vi "AIM 664 test Find Disabled Custom Device.vi"(8 "error in":errorcluster, 11 "TestCase in":refnum<class "AIM 664 Scripting.lvclass">) -> (0 "error out":errorcluster, 3 "TestCase out":refnum<class "AIM 664 Scripting.lvclass">)   [LabVIEW 2020, in "AIM 664 Scripting.lvclass"]
uses:
  AIM 664 Scripting.lvclass
  C:/Program Files (x86)/National Instruments/LabVIEW 2020/vi.lib/NI/VeriStand Custom Device Testing Tools/VeriStandScriptingTestCase/VeriStandScriptingTestCase.lvclass
  <vilib>/NI/VeriStand Custom Device Testing Tools/VeriStandScriptingTestCase/VeriStandScriptingTestCase.lvclass/VeriStandScriptingTestCase.ctl
  <vilib>/NI/VeriStand Custom Device Testing Tools/VeriStandScriptingTestCase/Read Target.vi
  NationalInstruments.VeriStand.SystemDefinitionAPI
  <vilib>/addons/_JKI Toolkits/VI Tester/TestCase.llb/TestCase.lvclass
  Scripting/AIM ARINC 664 Scripting.lvlib
  C:/Program Files (x86)/National Instruments/LabVIEW 2020/vi.lib/addons/_JKI Toolkits/VI Tester/TestCase.llb/TestCase.lvclass
  C:/repos/niveristand-aim-arinc664-custom-device/Source/Custom Device Support/Tests/Unit/Scripting/AIM 664 Scripting.lvclass
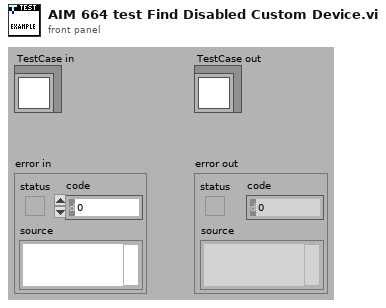
[diagram p1: front panel]
types:
  T1 = typedef "Custom Device API.lvlib/Custom Device Item Ref.ctl" = u64
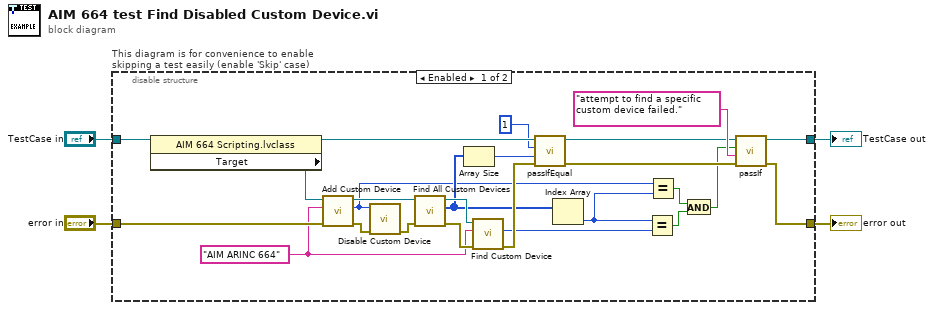
[diagram p0: block diagram]
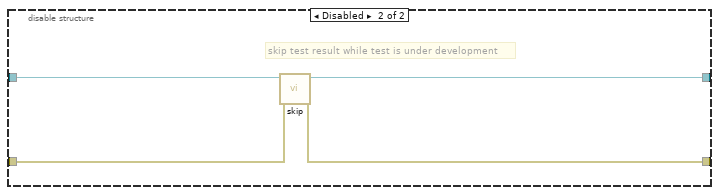
[diagram p2: hidden frame]
diagram:
  n1 = disable-structure "This diagram is for convenience to enable skipping a test easily (enable 'Skip' case)" shown="Enabled" {
    disable-tunnel: "TestCase in" -> [w25 w33]
    disable-tunnel: [w24 w31] -> w1
    disable-tunnel: [w23 w32] -> w3
    disable-tunnel: "error in" -> [w28 w30]
    frame Enabled {
      w12 = "AIM ARINC 664" ("name")
      n2 = property class="AIM 664 Scripting.lvclass"(reference=w25) -> (reference out=w27:refnum<class "AIM 664 Scripting.lvclass">, "Target"=w22:refnum<k24>)  [unwired: 1 in, 1 out]
      n3 = call "Add Custom Device.vi"("error in"=w28, "name"=w12, "target in"=w22) -> ("error out"=w21:errorcluster, "custom device"=w5:T1, "target out"=w17:refnum<k24>)  [unwired: 6 in]
      n4 = call "Disable Custom Device.vi"("error in"=w21, "custom device ref in"=w5) -> ("error out"=w16:errorcluster)  [unwired: 8 in, 1 out]
      n5 = call "Find All Custom Devices.vi"("error in"=w16, "target in"=w17) -> ("error out"=w15:errorcluster, "custom devices"=w8:u64[], "target out"=w13:refnum<k24>)  [unwired: 7 in]
      n6 = Array Size(array=w8) -> (size(s)=w18:i32)
      n7 = call "Find Custom Device.vi"("error in"=w15, "name"=w12, "target in"=w13) -> ("error out"=w14:errorcluster, "custom device"=w7:u64)  [unwired: 6 in, 1 out]
      n8 = call-dynamic "passIfEqual.vi"("error in (no error)"=w14, "y"=w18, "x"=1 ("disabled custom device"), "TestCase in"=w27) -> ("error out"=w20:errorcluster, "TestCase out"=w26:refnum<class "AIM 664 Scripting.lvclass">)  [unwired: 6 in]
      n9 = Index Array(array=w8) -> (element=w11:u64)  [unwired: 1 in]
      n10 = Equal?(x=w11, y=w7) -> (x = y?=w10:bool)
      n11 = Equal?(x=w5, y=w11) -> (x = y?=w9:bool)
      n12 = And(x=w9, y=w10) -> (x .and. y?=w6:bool)
      n13 = call-dynamic "passIf.vi"("error in (no error)"=w20, "message (\"\")"="attempt to find a specific custom device failed." ("message (\"\")"), "pass"=w6, "TestCase in"=w26) -> ("error out"=w23:errorcluster, "TestCase out"=w24:refnum<class "AIM 664 Scripting.lvclass">)  [unwired: 6 in]
    }
    frame Disabled {
      # "skip test result while test is under development"
      n14 = call <vilib>:"skip.vi"("error in (no error)"=w30, "TestCase in"=w33) -> ("error out"=w32:errorcluster, "TestCase out"=w31:refnum<class "AIM 664 Scripting.lvclass">)  [unwired: 8 in]
    }
  }
  "error out" <- w3
  "TestCase out" <- w1
